vi "ATF-Pump-Irms_Module_A.vi"(7 "Data FIFO Ref":T1, 8 "error in":errorcluster, 11 "TCP Network Connection in":refnum<k5>) -> (0 "error out":errorcluster, 3 "TCP Network Connection out":refnum<k5>)   [LabVIEW 2022 SP3]
uses:
  RT Controls/ATF-Pump-Data FIFO.ctl
  <vilib>/Analysis/3filter.llb/Filter Passband Type.ctl
  RT Controls/ATF-Pump-FGV Read write.ctl
  <vilib>/Analysis/NI_AALBase.lvlib
  <vilib>/ptbypt/NI_PtbyPt.lvlib
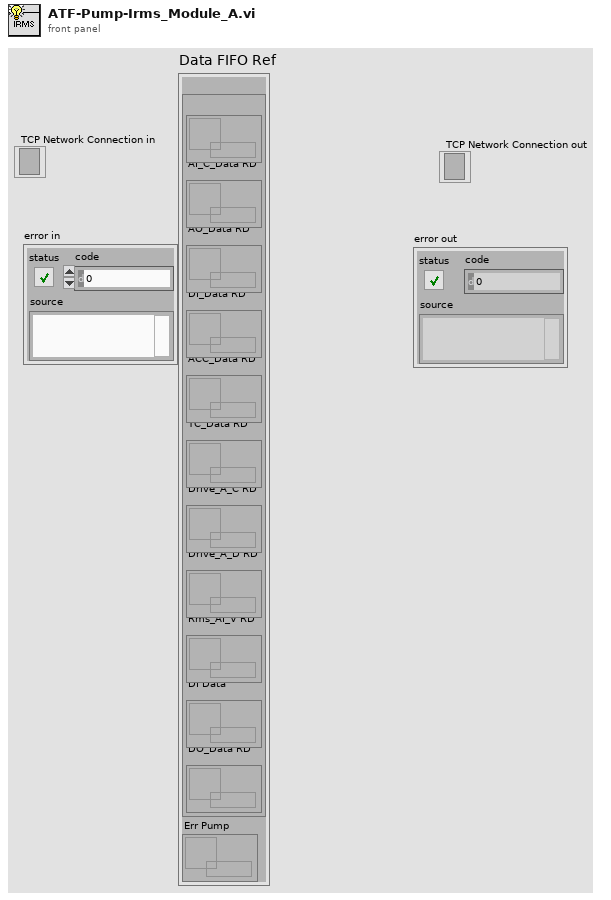
[diagram p1: front panel]
types:
  T1 = typedef "ATF-Pump-Data FIFO.ctl" = cluster{"RD":cluster{"AI_V_Data RD":refnum<queue>, "AI_C_Data RD":refnum<queue>, "AO_Data RD":refnum<queue>, "DI_Data RD":refnum<queue>, "ACC_Data RD":refnum<queue>, "TC_Data RD":refnum<queue>, "Drive_A_C RD":refnum<queue>, "Drive_A_D RD":refnum<queue>, "Rms_AI_V RD":refnum<queue>, "DI Data":refnum<queue>, "DO_Data RD":refnum<queue>}, "Err Pump":refnum<queue>}
  T2 = typedef "ATF-Pump-FGV Read write.ctl" = enum16{"Write", "Read"}
  T3 = cluster{"En_Drive_A":bool, "En_Drive_L":bool, "Exit_Drive_A":bool, "Exit_Drive_L":bool}
  T4 = typedef "NI_AALBase.lvlib/Filter Passband Type.ctl" = enum32{"Lowpass", "Highpass", "Bandpass", "Bandstop"}
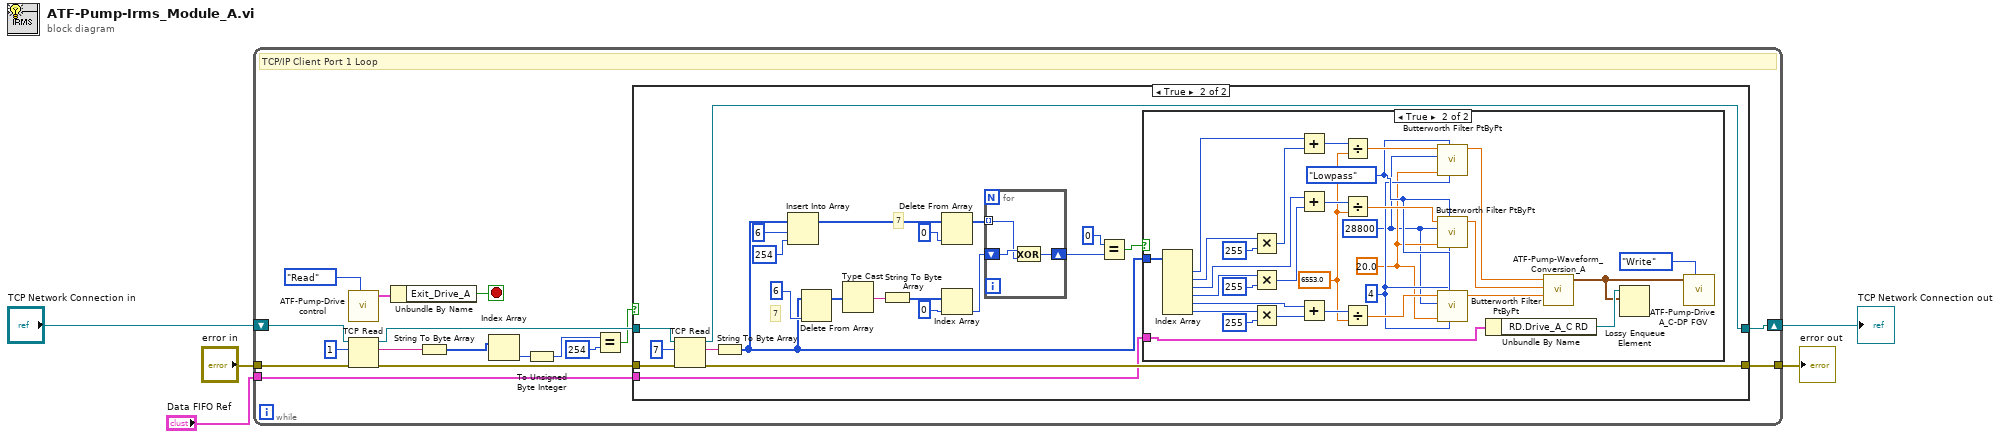
[diagram p0: block diagram]
diagram:
  n1 = while {
    tunnel: [w14] -> w3
    shift-right: [w13] -> w4
    shift-left: "TCP Network Connection in" -> [w22]
    tunnel: "error in" -> [w10]
    tunnel: "Data FIFO Ref" -> [w6]
    stop <- w8 stop-if-true
    # "TCP/IP Client Port 1 Loop"
    n2 = call "ATF-Pump-Drive control.vi"("Action"=enum16{"Init", "Write", "Read"}."Read") -> ("Loop Control Out"=w9:T3)  [unwired: 9 in, 1 out]
    n3 = TCP Read(connection ID=w22, bytes to read=1, error in (no error)=w10) -> (connection ID out=w15:refnum<k5>, data out=w16:string, error out=w11:errorcluster)  [unwired: 2 in]
    n4 = Unbundle By Name(w9) -> ("Exit_Drive_A"=w8:bool)
    n5 = String To Byte Array(string=w16) -> (unsigned byte array=w20:u8[])
    n6 = Index Array(array=w20) -> (element=w19:u8)  [unwired: 1 in]
    n7 = To Unsigned Byte Integer(number=w19) -> (unsigned 8bit integer=w18:u8)
    n8 = Equal?(x=w18, y=u8 254) -> (x = y?=w12:bool)
    n9 = case shown="True" w12 {
      tunnel: w15 -> [w23 w46]
      tunnel: w11 -> [w24 w45]
      tunnel: [w24 w44] -> w14
      tunnel: [w23 w43] -> w13
      tunnel: w6 -> [_ w25]
      frame False {
      }
      frame True {
        # "7"
        # "7"
        n10 = TCP Read(connection ID=w46, bytes to read=7, error in (no error)=w45) -> (connection ID out=w43:refnum<k5>, data out=w42:string, error out=w44:errorcluster)  [unwired: 2 in]
        n11 = String To Byte Array(string=w42) -> (unsigned byte array=w29:u8[])
        n12 = Insert Into Array(array=w29, index=6, new element=u8 254 ("new element/subarray")) -> (w30:u8[])
        n13 = Delete From Array(array=w29, index=6) -> (array with subset deleted=w33:u8[])  [unwired: 1 in, 1 out]
        n14 = Type Cast(x=w33) -> (*(type *) &x=w39:string)  [unwired: 1 in]
        n15 = String To Byte Array(string=w39) -> (unsigned byte array=w34:u8[])
        n16 = Delete From Array(array=w30, index=0) -> (array with subset deleted=w36:u8[])  [unwired: 1 in, 1 out]
        n17 = Index Array(array=w34, index=0) -> (element=w37:u8)
        n18 = for {
          shift-right: [w79] -> w27
          shift-left: w37 -> [w80]
          tunnel: w36 -> [w78] mode=indexing
          n19 = Exclusive Or(1:w78, 2:w80) -> (0:w79:u8)
        }
        n20 = Equal?(x=u8 0, y=w27) -> (x = y?=w26:bool)
        n21 = case shown="True" w26 {
          tunnel: w29 -> [_ w62]
          tunnel: w25 -> [_ w50]
          frame False {
          }
          frame True {
            w57 = Filter_Passband_Type."Lowpass" ("filter type")
            w56 = 4 ("order")
            w55 = 20.0 ("low cutoff freq: fl")
            w54 = 28800 ("rank")
            w61 = 6553.0
            n22 = Index Array(array=w62) -> (element #1=w75:u8, element #2=w74:u8, element #3=w69:u8, element #4=w68:u8, element #5=w67:u8, element #6=w66:u8)  [unwired: 6 in]
            n23 = Multiply(x=w74, y=u32 255) -> (x*y=w76:u32)
            n24 = Multiply(x=w68, y=u32 255) -> (x*y=w73:u32)
            n25 = Multiply(x=w66, y=u32 255) -> (x*y=w70:u32)
            n26 = Add(x=w75, y=w76) -> (x+y=w65:u32)
            n27 = Add(x=w69, y=w73) -> (x+y=w64:u32)
            n28 = Add(x=w67, y=w70) -> (x+y=w63:u32)
            n29 = Divide(x=w65, y=w61) -> (x/y=w60:dbl)
            n30 = Divide(x=w64, y=w61) -> (x/y=w59:dbl)
            n31 = Divide(x=w63, y=w61) -> (x/y=w58:dbl)
            n32 = call <vilib>:"Butterworth Filter PtByPt.vi"("order"=w56, "filter type"=w57, "low cutoff freq: fl"=w55, "sampling freq: fs"=w54, "x"=w60) -> ("Filtered x"=w53:dbl)  [unwired: 4 in, 1 out]
            n33 = call <vilib>:"Butterworth Filter PtByPt.vi"("order"=w56, "filter type"=w57, "low cutoff freq: fl"=w55, "sampling freq: fs"=w54, "x"=w59) -> ("Filtered x"=w52:dbl)  [unwired: 4 in, 1 out]
            n34 = call <vilib>:"Butterworth Filter PtByPt.vi"("order"=w56, "filter type"=w57, "low cutoff freq: fl"=w55, "sampling freq: fs"=w54, "x"=w58) -> ("Filtered x"=w51:dbl)  [unwired: 4 in, 1 out]
            n35 = Unbundle By Name(w50) -> ("RD.Drive_A_C RD"=w49:refnum<queue>)
            n36 = call "ATF-Pump-Waveform_Conversion_A.vi"("Irms3"=w51, "Irms2"=w52, "Irms1"=w53) -> ("Array"=w47:waveform(dbl)[])  [unwired: 8 in]
            n37 = Lossy Enqueue Element(queue=w49, element=w47) -> ()  [unwired: 1 in, 4 out]
            n38 = call "ATF-Pump-Drive A_C-DP FGV.vi"("Write/Read"=ATF-Pump-FGV_Read_write."Write", "Drive A_C"=w47) -> ()  [unwired: 8 in, 2 out]
          }
        }
      }
    }
  }
  "TCP Network Connection out" <- w4
  "error out" <- w3
